vi "Write_Enviroment_Register.vi"(0 "Intervalo Temperatura":u16, 1 "Intervalo Presion":u16, 2 "Intervalo Humedad":u16, 3 "Intervalo Color":u16, 4 "Modo Aire":u8, 5 "Intensidad Rojo":u8, 6 "Intensidad Verde":u8, 7 "Intensidad Azul":u8, 8 "COM Bluegiga in":refnum<visa-resource-name>, 9 "error in (no error)":errorcluster, 11 "Handle table":string[][](array[string]), 12 "Service UUID":string, 15 "Connection Status":T1={"MAC Address"="", "cnx handle"=0, "cnx flags"=0, "Address Type"=125, "Connection Interval (ms)"=125, "Timeout(ms)"=125, "Latency"=0, "bonding handle"=0} {"Address Type" items=["Public", "Random"]}, 16 "Characteristic UUID":string) -> (20 "COM Bluegiga out":refnum<visa-resource-name>, 27 "error out":errorcluster)   [LabVIEW 2020]
uses:
  <vilib>/BLE/type_def/connection_status_bundle.ctl
  <vilib>/BLE/type_def/address_type.ctl
  <vilib>/BLE/ble_functions/ble_write_by_service_characteristic_uint8array.vi
panel:
  out "output array":u8[](array[numeric])
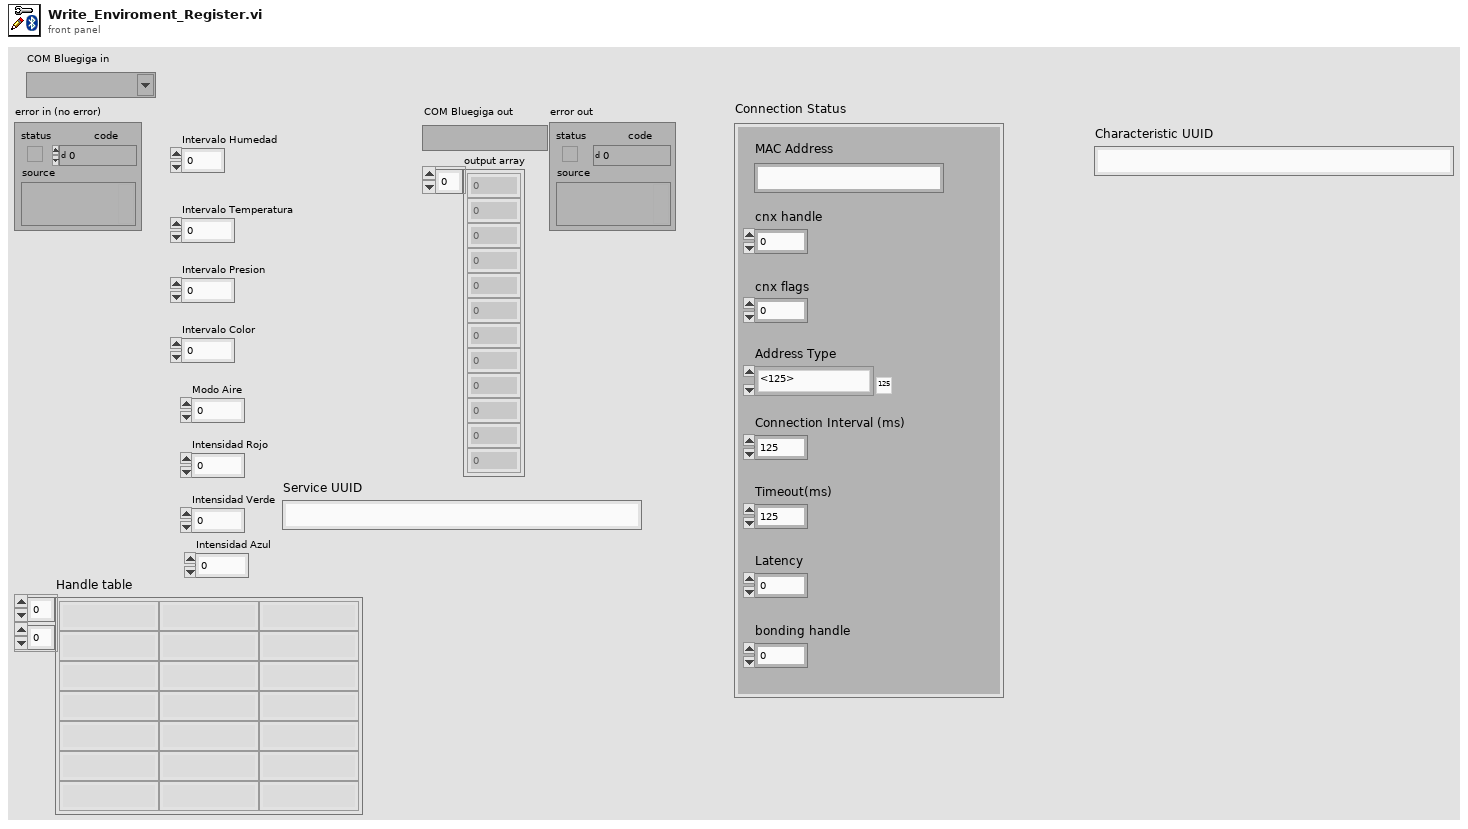
[diagram p1: front panel]
types:
  T1 = typedef "connection_status_bundle.ctl" = cluster{"MAC Address":string, "cnx handle":u8, "cnx flags":u8, "Address Type":T2, "Connection Interval (ms)":u16, "Timeout(ms)":u16, "Latency":u16, "bonding handle":u8}
  T2 = typedef "address_type.ctl" = u8
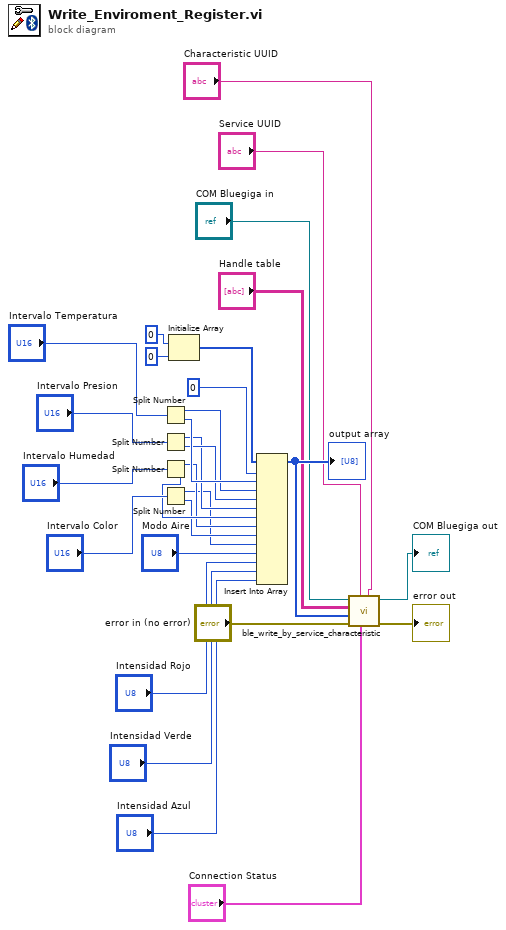
[diagram p0: block diagram]
diagram:
  n1 = Split Number(x="Intervalo Temperatura") -> (hi(x)=w7:u8, lo(x)=w8:u8)
  n2 = Split Number(x="Intervalo Presion") -> (hi(x)=w5:u8, lo(x)=w6:u8)
  n3 = Split Number(x="Intervalo Humedad") -> (hi(x)=w3:u8, lo(x)=w4:u8)
  n4 = Split Number(x="Intervalo Color") -> (hi(x)=w1:u8, lo(x)=w2:u8)
  n5 = Initialize Array(u8 0 ("element"), 0 ("dimension size")) -> (w25:u8[])
  n6 = Insert Into Array(array=w25, index=0, new element #1=w8, new element #2=w7, new element #3=w6, new element #4=w5, new element #5=w4, new element #6=w3, new element #7=w2, new element #8=w1, new element #9="Modo Aire", new element #10="Intensidad Rojo", new element #11="Intensidad Verde", new element #12="Intensidad Azul") -> (w17:u8[])
  "output array" <- w17
  n7 = call-poly <vilib>:"ble_write_by_service_characteristic.vi"("Characteristic UUID"="Characteristic UUID", "Connection Status"="Connection Status", "Service UUID"="Service UUID", "error in (no error)"="error in (no error)", "data"=w17, "Handle table"="Handle table", "COM Bluegiga in"="COM Bluegiga in") -> ("error out"=→"error out":errorcluster, "COM Bluegiga out"=→"COM Bluegiga out":refnum<visa-resource-name>)  [unwired: 3 in]
